vi "credit update.vi"(8 "error in (no error)":errorcluster, 10 "Credito":dbl, 11 "UI Actor in":refnum<class "UI Actor.lvclass">) -> (0 "error out":errorcluster, 3 "UI Actor out":refnum<class "UI Actor.lvclass">)   [LabVIEW 2019, in "UI Actor.lvlib" / "UI Actor.lvclass"]
uses:
  UI Actor.lvclass
  UI Actor.lvclass/UI Actor.ctl
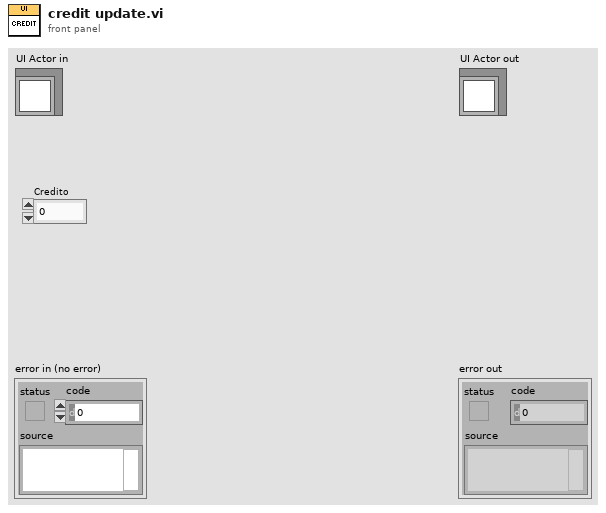
[diagram p1: front panel]
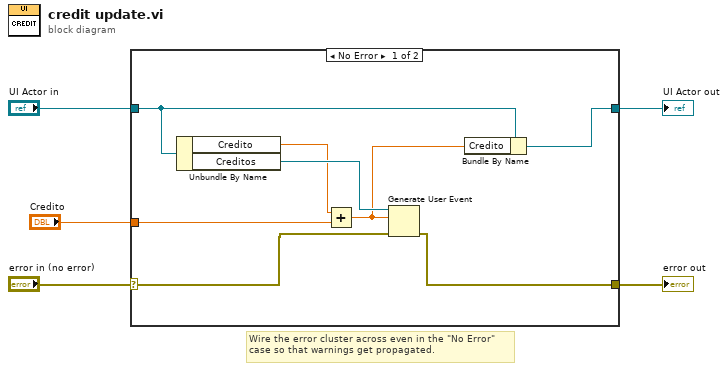
[diagram p0: block diagram]
diagram:
  # "Wire the error cluster across even in the \"No Error\"\ncase so that warnings get propagated."
  n1 = case shown="No Error" "error in (no error)" {
    selector: "error in (no error)" -> [w12 w15]
    tunnel: [w11 w15] -> w4
    tunnel: [w9 w14] -> w2
    tunnel: "UI Actor in" -> [w10 w14]
    tunnel: "Credito" -> [w7 _]
    frame No Error {
      n2 = Unbundle By Name(w10) -> ("Credito"=w8:dbl, "Creditos"=w13:refnum<user-event>)
      n3 = Add(x=w8, y=w7) -> (x+y=w6:dbl)
      n4 = Generate User Event(user event=w13, event data cluster=w6, error in=w12) -> (error out=w11:errorcluster)  [unwired: 1 in, 1 out]
      n5 = Bundle By Name(cluster=w10, "Credito"=w6) -> (w9:refnum<class "UI Actor.lvclass">)
    }
    frame Error {
    }
  }
  "error out" <- w4
  "UI Actor out" <- w2
